vi "ief_get_single_output.vi"(3 "error in (no error)":errorcluster, 4 "Single Output Number":u16=1 min=1 max=1024, 5 "Tagprefix in":refnum<k21>) -> (0 "error out (no error)":errorcluster, 1 "Single Output State":bool, 2 "Tagprefix out":refnum<k21>)   [LabVIEW 2015, in "IEF Werner.lvlib"]
doc: "The VI returns the present single output state of the chosen single output.\n\nSingle Output Number Range:\n0001 - 0400, hex\n1 - 1024, dec"
uses:
  IEF Werner.lvlib
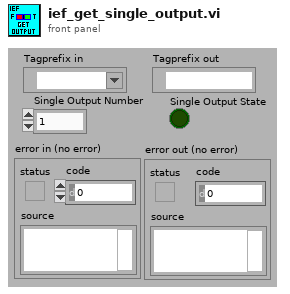
[diagram p1: front panel]
types:
  T1 = typedef "Semaphore RefNum" = refnum<k1>
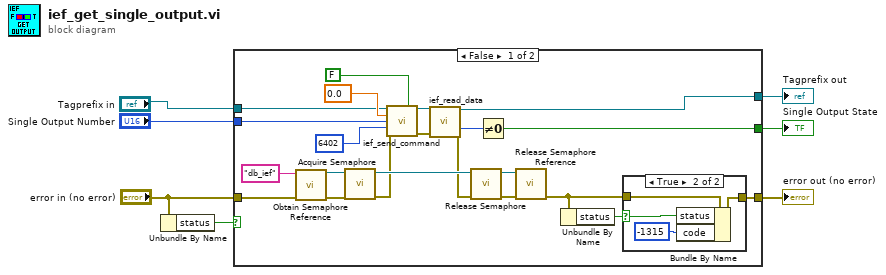
[diagram p0: block diagram]
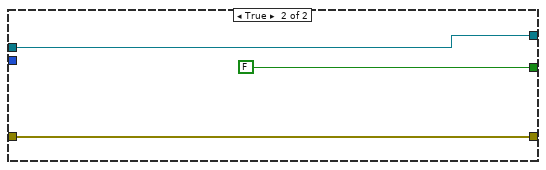
[diagram p3: hidden frame]
diagram:
  n1 = Unbundle By Name("error in (no error)") -> ("status"=w4:bool)
  n2 = case shown="False" w4 {
    tunnel: "Single Output Number" -> [w27 _]
    tunnel: "error in (no error)" -> [w15 w37]
    tunnel: [w25 w37] -> w6
    tunnel: [w22 FALSE] -> w3
    tunnel: "Tagprefix in" -> [w10 w36]
    tunnel: [w8 w36] -> w1
    frame False {
      n3 = call <vilib>:"Obtain Semaphore Reference.vi"("error in (no error)"=w15, "name (unnamed)"="db_ief") -> ("error out"=w19:errorcluster, "semaphore"=w20:T1)  [unwired: 3 in, 1 out]
      n4 = call <vilib>:"Acquire Semaphore.vi"("error in (no error)"=w19, "semaphore"=w20) -> ("error out"=w14:errorcluster, "semaphore out"=w18:T1)  [unwired: 3 in, 1 out]
      n5 = call "ief_send_command.vi"("Tagprefix in"=w10, "Command datum of type real"=FALSE, "Command datum"=sgl 0.0, "Command parameter"=w27, "Command code"=u16 6402, "error in (no error)"=w14) -> ("Tagprefix out"=w9:refnum<k21>, "error out (no error)"=w26:errorcluster)  [unwired: 4 in, 4 out]
      n6 = call "ief_read_data.vi"("Tagprefix in"=w9, "error in (no error)"=w26) -> ("Tagprefix out"=w8:refnum<k21>, "value uint 16"=w23:u16, "error out (no error)"=w13:errorcluster)  [unwired: 7 in, 4 out]
      n7 = call <vilib>:"Release Semaphore.vi"("error in (no error)"=w13, "semaphore"=w18) -> ("error out"=w17:errorcluster, "semaphore out"=w16:T1)  [unwired: 4 in]
      n8 = Not Equal To 0?(x=w23) -> (x != 0?=w22:bool)
      n9 = call <vilib>:"Release Semaphore Reference.vi"("error in (no error)"=w17, "semaphore"=w16) -> ("error out"=w12:errorcluster)  [unwired: 8 in, 1 out]
      n10 = Unbundle By Name(w12) -> ("status"=w24:bool)
      n11 = case shown="True" w24 {
        selector: w24 -> [_ w31]
        tunnel: [w30 w33] -> w25
        tunnel: w12 -> [w30 w34]
        frame False {
        }
        frame True {
          n12 = Bundle By Name(cluster=w34, "status"=w31, "code"=-1315) -> (w33:errorcluster)
        }
      }
    }
    frame True {
    }
  }
  "error out (no error)" <- w6
  "Single Output State" <- w3
  "Tagprefix out" <- w1
